vi "Motor PWM 2.vi"() -> ()   [LabVIEW 2017]
uses:
  <vilib>/myRIO/Instrument Drivers/Onboard IO/PWM/vis/Set Duty Cycle and Frequency.vi
  <vilib>/myRIO/Common/Instrument Driver Framework/myRIO v1.0/UART/vis/myRIO v1.0 Close UART.vi
  <vilib>/myRIO/Instrument Drivers/Onboard IO/PWM/vis/Smart Open.vi
  <vilib>/Utility/error.llb/Error Cluster From Error Code.vi
  <vilib>/myRIO/Common/Instrument Driver Framework/myRIO v1.0/PWM/vis/myRIO v1.0 Write PWM.vi
  <vilib>/myRIO/Common/Instrument Driver Framework/Utilities/vis/FPGA Ref Manager.vi
  <vilib>/myRIO/Common/Instrument Driver Framework/myRIO v1.0/myRIO v1.0 Reset FPGA.vi
  <vilib>/myRIO/Common/Instrument Driver Framework/myRIO v1.0/IRQ/vis/myRIO v1.0 IRQ Info FGV.vi
  <vilib>/myRIO/Common/Instrument Driver Framework/myRIO v1.0/IRQ/vis/myRIO v1.0 Timer IRQ Info FGV.vi
  <vilib>/myRIO/Common/Instrument Driver Framework/myRIO v1.0/IRQ/vis/myRIO v1.0 ISR Agent.vi
  <vilib>/myRIO/Instrument Drivers/Utilities/Utilities.lvlib
panel:
  in  "Nome do canal":tag="C/PWM0"
  in  "stop":bool
  in  "PWM freq [Hz]":dbl(slide)=100.0 scale=40.0..40000.0
  in  "PWM duty  [%]":dbl(slide) scale=0.0..100.0
  in  "Enable":bool
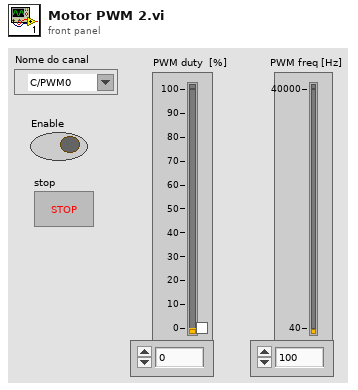
[diagram p1: front panel]
types:
  T1 = typedef "PWM.lvlib/PWM Reference.ctl" = cluster{"myRIO Reference":T2, "PWM Channels Enum":T6, "PWM Configuration":T7}
  T2 = typedef "myRIO Generic Hardware Reference.ctl" = cluster{"myRIO Model":T3, "myRIO Hardware Reference":T4}
  T3 = typedef "Hardware Version Enum.ctl" = enum16{"Unknown", "myRIO-1900", "myRIO-1950", "roboRIO", "NI ELVIS RIO CM"}
  T4 = typedef "myRIO v1.0 Reference.ctl" = cluster{"Generic FPGA Reference":T5, "Allow multiple opens":bool}
  T5 = typedef "Generic FPGA Reference.ctl" = refnum<k20>
  T6 = typedef "PWM Channels Enum.ctl" = enum16{"Not Connected", "C/PWM0", "C/PWM1", "A/PWM0", "A/PWM1", "A/PWM2", "B/PWM0", "B/PWM1", "B/PWM2", "PWM/PWM0", "PWM/PWM1", "PWM/PWM2", "PWM/PWM3", "PWM/PWM4", "PWM/PWM5", "PWM/PWM6", "PWM/PWM7", "PWM/PWM8", "PWM/PWM9"}
  T7 = typedef "PWM.lvlib/PWM Configuration.ctl" = cluster{"Frequency":dbl, "Duty Cycle":dbl}
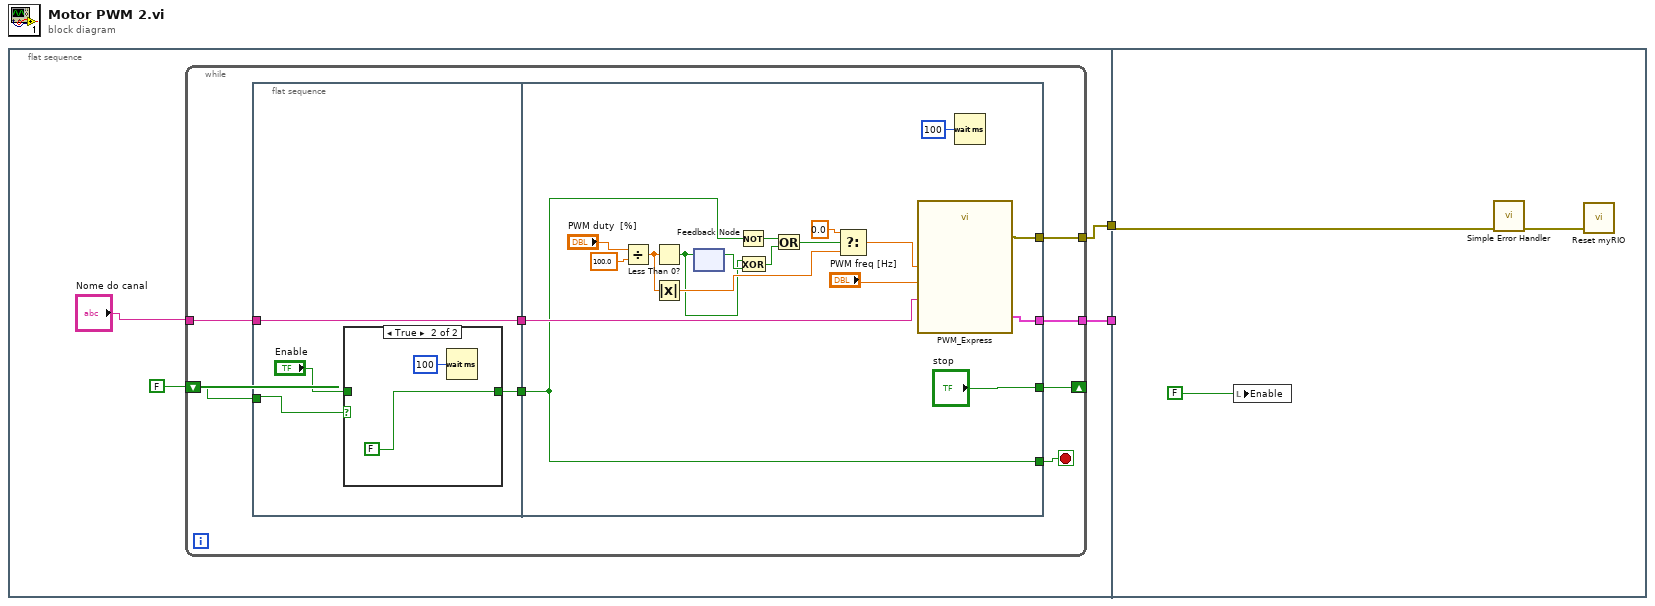
[diagram p0: block diagram]
diagram:
  n1 = flat-sequence {
    tunnel: [w6] -> w2
    tunnel: [w4] -> w1
    tunnel: w1 -> [_]
    tunnel: w2 -> [w41]
    frame #0 {
      n2 = while {
        tunnel: [w14] -> w6
        tunnel: "Nome do canal" -> [w13]
        tunnel: [w12] -> w4
        shift-right: [w11] -> _
        shift-left: FALSE ("stop") -> [w9]
        stop <- w7 stop-if-true
        n3 = flat-sequence {
          tunnel: w13 -> [w18]
          tunnel: [w18] -> w10
          tunnel: w9 -> [w17]
          tunnel: [w15] -> w8
          tunnel: [w28] -> w14
          tunnel: [w24] -> w12
          tunnel: ["stop"] -> w11
          tunnel: w10 -> [w25]
          tunnel: w8 -> [w22]
          tunnel: [w22] -> w7
          frame #0 {
            n4 = case shown="True" w17 {
              tunnel: "Enable" -> [w19 _]
              tunnel: [w19 FALSE] -> w15
              frame False {
              }
              frame True {
                n5 = Wait (ms)(milliseconds to wait=u32 100) -> ()  [unwired: 1 out]
              }
            }
          }
          frame #1 {
            n6 = Divide(x="PWM duty  [%]", y=100.0) -> (x/y=w32:dbl)
            n7 = Less Than 0?(x=w32) -> (x < 0?=w29:bool)
            n8 = Absolute Value(x=w32) -> (abs(x)=w31:dbl)
            n9 = feedback #1() -> (w38:bool)  [unwired: 1 in]
            n10 = feedback-in #1(w29) -> ()
            n11 = Not(x=w22) -> (.not. x?=w34:bool)
            n12 = Exclusive Or(1:w38, 2:w29) -> (0:w36:bool)
            n13 = Or(x=w34, y=w36) -> (x .or. y?=w35:bool)
            n14 = Select(t=0.0 ("f"), s=w35, f=w31) -> (s? t:f=w26:dbl)
            n15 = call "PWM_Express.vi"("Channel Name"=w25, "Frequency [Hz]"="PWM freq [Hz]", "Duty Cycle"=w26) -> ("error out"=w28:errorcluster, "PWM Ref Out"=w24:T1)  [unwired: 3 in]
            n16 = Wait (ms)(milliseconds to wait=u32 100) -> ()  [unwired: 1 out]
          }
        }
      }
    }
    frame #1 {
      n17 = local write "Enable"(FALSE) -> ()
      n18 = call <vilib>:"Simple Error Handler.vi"("error in (no error)"=w41) -> ("error out"=w42:errorcluster)  [unwired: 4 in, 4 out]
      n19 = call <vilib>:"Reset myRIO.vi"("error in (no error)"=w42) -> ()  [unwired: 10 in, 1 out]
    }
  }
